vi "Read Z_State.vi"(11 "valve_VCH_Z_state in":refnum<class "valve_VCH_Z_state.lvclass">) -> (2 "Z_State_VCH":T1=enum."on min", 3 "valve_VCH_Z_state out":refnum<class "valve_VCH_Z_state.lvclass">)   [LabVIEW 2019, in "valve_VCH_Z_state.lvclass"]
uses:
  valve_VCH_Z_state.lvclass
  ctl/Z_State_VCH.ctl
  valve_VCH_Z_state.lvclass/valve_VCH_Z_state.ctl
  Valves.lvlib
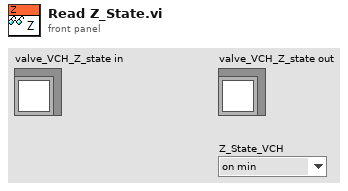
[diagram p1: front panel]
types:
  T1 = typedef "Valves.lvlib/Z_State_VCH.ctl" = enum8{"initialization", "alarm", "disabled", "not ready", "closed ready", "reserv", "reserv1", "reserv2", "reserv3", "check", "on min", "open", "on (closed)"}
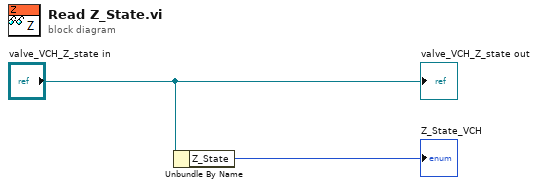
[diagram p0: block diagram]
diagram:
  n1 = Unbundle By Name("valve_VCH_Z_state in") -> ("Z_State"=→"Z_State_VCH":T1)
  "valve_VCH_Z_state out" <- "valve_VCH_Z_state in"
